vi "Configure Measurement Cursors.vi"(11 "State in":T1={"Graph Visible Items"={"Plot Legend"=FALSE, "Scale Legend"=FALSE, "Graph Palette"=FALSE, "Cursor Legend"=FALSE, "X Scrollbar"=FALSE}, "View Table"=FALSE, "Table Visible Items"={"Vertical Scrollbar"=FALSE, "Horizontal Scrollbar"=FALSE, "Row Headers"=FALSE, "Column Headers"=FALSE, "Vertical Lines"=FALSE, "Horizontal Lines"=FALSE}, "Header Font"={"Font Name"="", "Size"=0, "Bold"=FALSE, "Italic"=FALSE, "Underline"=FALSE, "Strikeout"=FALSE, "Color"=0}, "Cell Font"={"Font Name"="", "Size"=0, "Bold"=FALSE, "Italic"=FALSE, "Underline"=FALSE, "Strikeout"=FALSE, "Color"=0}, "Description and Tip..."={"Description"="", "Tip"=""}, "Moveable Splitter Position"=0, "Measurement Cursor Configuration"={"XY"={"enable XY"=FALSE, "Position (X)"=[], "Type"=enum."Absolute", "Y reference"=0.0, "color"=0}, "band"={"enable band"=FALSE, "B1"=0.0, "B2"=0.0, "Fixed bandwidth (B2-B1)"=0.0, "B1 color"=0, "B2 color"=0}, "harmonic"={"enable harmonics"=FALSE, "X reference (1X)"=0.0, "Maximum"=0, "Subset"=enum."All", "1X color"=0, "MX color"=0}, "sideband"={"enable sideband"=FALSE, "X center (C)"=0.0, "Sidebands"=0, "X spacing (s)"=0.0, "Center color"=0, "Sideband color"=0}}, "Cursors"={"List"=[], "Tags"=[]}, "X Increment"=0.0, "X Scale"={"Label Visible"=FALSE, "Label Text"="", "Mapping Mode"=0, "Format String"=""}, "Y Scale"={"Label Visible"=FALSE, "Label Text"="", "Mapping Mode"=0, "Format String"=""}, "Colors"={"background"=16777215, "major grid"=8355711, "minor grid"=12632256, "font"=0}, "desired spectrum view"={"scaling"={"linear/dB"=enum."no change", "dB reference"=0.0, "power/magnitude"=enum."no change", "view"=enum."no change"}, "spectral density"=enum."no change"}, "Plot Color Wheel"=[3381759, 32768, 982784, 4375295, 13827953, 13457919, 16757522, 4343295, 16728758, 12095254], "Plots"=[], "registered user events"=variant, "Lock 1X to Peak"=FALSE, "spectrum component"=32, "phase spectrum view"={"desired units"=0, "desired wrapping"=4}} caption="State" {"phase spectrum view"."desired wrapping" items=["No change", "Unwrap", "Wrap: -360 to 0", "Wrap: -270 to 90", "Wrap: -180 to 180", "Wrap: -90 to 270", "Wrap: 0 to 360", "Wrap: custom range"]; "phase spectrum view"."desired units" items=["No change", "Radians", "Degrees", "Cycles"]; "spectrum component" items=["Magnitude^2"=37, "Magnitude"=32, "Phase"=33, "Real"=34, "Imaginary"=35, "Coherence"=36, "Unknown"=99]; "Y Scale"."Mapping Mode" items=["Linear", "Logarithmic", "dB"]; "X Scale"."Mapping Mode" items=["Linear", "Logarithmic"]}) -> (1 "OK":bool, 3 "State out":T1={"Graph Visible Items"={"Plot Legend"=FALSE, "Scale Legend"=FALSE, "Graph Palette"=FALSE, "Cursor Legend"=FALSE, "X Scrollbar"=FALSE}, "View Table"=FALSE, "Table Visible Items"={"Vertical Scrollbar"=FALSE, "Horizontal Scrollbar"=FALSE, "Row Headers"=FALSE, "Column Headers"=FALSE, "Vertical Lines"=FALSE, "Horizontal Lines"=FALSE}, "Header Font"={"Font Name"="", "Size"=0, "Bold"=FALSE, "Italic"=FALSE, "Underline"=FALSE, "Strikeout"=FALSE, "Color"=0}, "Cell Font"={"Font Name"="", "Size"=0, "Bold"=FALSE, "Italic"=FALSE, "Underline"=FALSE, "Strikeout"=FALSE, "Color"=0}, "Description and Tip..."={"Description"="", "Tip"=""}, "Moveable Splitter Position"=0, "Measurement Cursor Configuration"={"XY"={"enable XY"=FALSE, "Position (X)"=[], "Type"=enum."Absolute", "Y reference"=0.0, "color"=0}, "band"={"enable band"=FALSE, "B1"=0.0, "B2"=0.0, "Fixed bandwidth (B2-B1)"=0.0, "B1 color"=0, "B2 color"=0}, "harmonic"={"enable harmonics"=FALSE, "X reference (1X)"=0.0, "Maximum"=0, "Subset"=enum."All", "1X color"=0, "MX color"=0}, "sideband"={"enable sideband"=FALSE, "X center (C)"=0.0, "Sidebands"=0, "X spacing (s)"=0.0, "Center color"=0, "Sideband color"=0}}, "Cursors"={"List"=[], "Tags"=[]}, "X Increment"=0.0, "X Scale"={"Label Visible"=FALSE, "Label Text"="", "Mapping Mode"=0, "Format String"=""}, "Y Scale"={"Label Visible"=FALSE, "Label Text"="", "Mapping Mode"=0, "Format String"=""}, "Colors"={"background"=16777215, "major grid"=8355711, "minor grid"=12632256, "font"=0}, "desired spectrum view"={"scaling"={"linear/dB"=enum."no change", "dB reference"=0.0, "power/magnitude"=enum."no change", "view"=enum."no change"}, "spectral density"=enum."no change"}, "Plot Color Wheel"=[3381759, 32768, 982784, 4375295, 13827953, 13457919, 16757522, 4343295, 16728758, 12095254], "Plots"=[], "registered user events"=variant, "Lock 1X to Peak"=FALSE, "spectrum component"=32, "phase spectrum view"={"desired units"=0, "desired wrapping"=4}} caption="State" {"phase spectrum view"."desired wrapping" items=["No change", "Unwrap", "Wrap: -360 to 0", "Wrap: -270 to 90", "Wrap: -180 to 180", "Wrap: -90 to 270", "Wrap: 0 to 360", "Wrap: custom range"]; "phase spectrum view"."desired units" items=["No change", "Radians", "Degrees", "Cycles"]; "spectrum component" items=["Magnitude^2"=37, "Magnitude"=32, "Phase"=33, "Real"=34, "Imaginary"=35, "Coherence"=36, "Unknown"=99]; "Y Scale"."Mapping Mode" items=["Linear", "Logarithmic", "dB"]; "X Scale"."Mapping Mode" items=["Linear", "Logarithmic"]})   [LabVIEW 2017, in "Spectrum with Cursors.xctl"]
doc: "Dialog for cursor configuration."
uses:
  <vilib>/addons/_XControls/Spectrum with Cursors/Spectrum with Cursors.xctl
  <vilib>/addons/_XControls/Spectrum with Cursors/Controls/State.ctl
  <vilib>/Utility/miscctls.llb/LVFontTypeDef.ctl
  <vilib>/addons/_XControls/Spectrum with Cursors/Controls/Measurement Cursor Configuration.ctl
  <vilib>/addons/_NISVFA/_Shared subVIs/Controls/NI Spectrum Component.ctl
panel:
  in  "XY color":u32(colorbox)
  in  "enable XY":bool
  in  "Type":enum16{"Absolute", "Relative"}(ring)
  in  "Position (i)":dbl[](array[numeric]) min=0.0 step=1.0
  in  "Y reference":dbl
  in  "B2 color":u32(colorbox)
  in  "B1 color":u32(colorbox)
  in  "Fixed bandwidth (B2-B1)":dbl=-1.0 caption="Fixed bandwidth"
  in  "enable band":bool
  in  "Stop (b2)":dbl=480.0
  in  "Start (b1)":dbl=20.0
  in  "1X color":u32(colorbox)
  in  "MX color":u32(colorbox)
  in  "enable harmonics":bool
  in  "Maximum (mX)":i32=10 min=2 max=99 step=1
  in  "X reference (1X)":dbl=60.0 min=0.001 step=1.0
  in  "Subset":enum16{"All", "Even", "Odd"}(ring)
  in  "Center color":u32(colorbox)
  in  "Sideband color":u32(colorbox)
  in  "Sidebands (sn)":i32=2 min=1 max=9 step=1
  in  "enable sideband":bool
  in  "X spacing (s)":dbl=60.0 min=0.0 step=1.0
  in  "X center (C)":dbl=8000.0 min=0.001 step=0.001
  in  "Cancel":bool
  in  "OK":bool
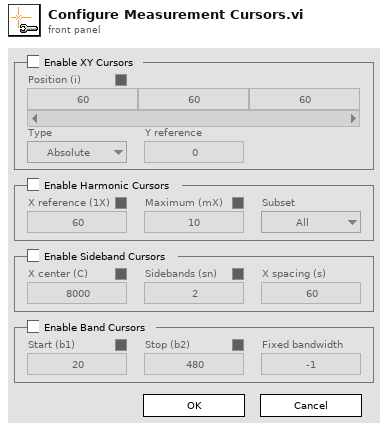
[diagram p1: front panel]
types:
  T1 = typedef "Spectrum with Cursors.xctl/State.ctl" = cluster{"Graph Visible Items":cluster{"Plot Legend":bool, "Scale Legend":bool, "Graph Palette":bool, "Cursor Legend":bool, "X Scrollbar":bool}, "View Table":bool, "Table Visible Items":cluster{"Vertical Scrollbar":bool, "Horizontal Scrollbar":bool, "Row Headers":bool, "Column Headers":bool, "Vertical Lines":bool, "Horizontal Lines":bool}, "Header Font":T2, "Cell Font":T2, "Description and Tip...":cluster{"Description":string, "Tip":string}, "Moveable Splitter Position":i32, "Measurement Cursor Configuration":T3, "Cursors":cluster{"List":cluster{"Name":string, "Color":u32, "Style":i32, "Point Style":u8, "Name Visible":bool, "Allow Drag":bool, "Cursor Mode":u32, "Plot":i32, "Index":i32, "Position":cluster{"X":dbl, "Y":dbl}, "X Scale":u32, "Y Scale":u32, "Watch Plots":i32[], "Watch All Plots":bool, "Plot Area":i32, "Label Offset":cluster{"X":dbl, "Y":dbl}}[], "Tags":variant[]}, "X Increment":dbl, "X Scale":cluster{"Label Visible":bool, "Label Text":string, "Mapping Mode":u8, "Format String":string}, "Y Scale":cluster{"Label Visible":bool, "Label Text":string, "Mapping Mode":u8, "Format String":string}, "Colors":cluster{"background":u32, "major grid":u32, "minor grid":u32, "font":u32}, "desired spectrum view":cluster{"scaling":cluster{"linear/dB":enum16{"no change", "linear", "dB"}, "dB reference":dbl, "power/magnitude":enum16{"no change", "power", "magnitude"}, "view":enum16{"no change", "rms", "peak", "peak-peak"}}, "spectral density":enum16{"no change", "spectrum", "spectral density"}}, "Plot Color Wheel":u32[], "Plots":cluster{"Name":string, "Line Color":u32, "Line Style":u8, "Line Width":u8, "Fill/Point Color":u32, "Point Style":u8, "Fill To":i16, "Interpolation":u8, "Anti-aliased":bool}[], "registered user events":variant, "Lock 1X to Peak":bool, "spectrum component":T4, "phase spectrum view":cluster{"desired units":u16, "desired wrapping":u16}}
  T2 = typedef "LVFontTypeDef.ctl" = cluster{"Font Name":string, "Size":u16, "Bold":bool, "Italic":bool, "Underline":bool, "Strikeout":bool, "Color":u32}
  T3 = typedef "Spectrum with Cursors.xctl/Measurement Cursor Configuration.ctl" = cluster{"XY":cluster{"enable XY":bool, "Position (X)":dbl[], "Type":enum16{"Absolute", "Relative"}, "Y reference":dbl, "color":u32}, "band":cluster{"enable band":bool, "B1":dbl, "B2":dbl, "Fixed bandwidth (B2-B1)":dbl, "B1 color":u32, "B2 color":u32}, "harmonic":cluster{"enable harmonics":bool, "X reference (1X)":dbl, "Maximum":i32, "Subset":enum16{"All", "Even", "Odd"}, "1X color":u32, "MX color":u32}, "sideband":cluster{"enable sideband":bool, "X center (C)":dbl, "Sidebands":i32, "X spacing (s)":dbl, "Center color":u32, "Sideband color":u32}}
  T4 = typedef "NI Spectrum Component.ctl" = u16
  T5 = cluster{"enable XY":bool, "Position (X)":dbl[], "Type":enum16{"Absolute", "Relative"}, "Y reference":dbl, "color":u32}
  T6 = cluster{"enable harmonics":bool, "X reference (1X)":dbl, "Maximum":i32, "Subset":enum16{"All", "Even", "Odd"}, "1X color":u32, "MX color":u32}
  T7 = cluster{"enable sideband":bool, "X center (C)":dbl, "Sidebands":i32, "X spacing (s)":dbl, "Center color":u32, "Sideband color":u32}
  T8 = cluster{"enable band":bool, "B1":dbl, "B2":dbl, "Fixed bandwidth (B2-B1)":dbl, "B1 color":u32, "B2 color":u32}
  T9 = enum8{"Enabled", "Disabled", "Disabled and Grayed Out"}
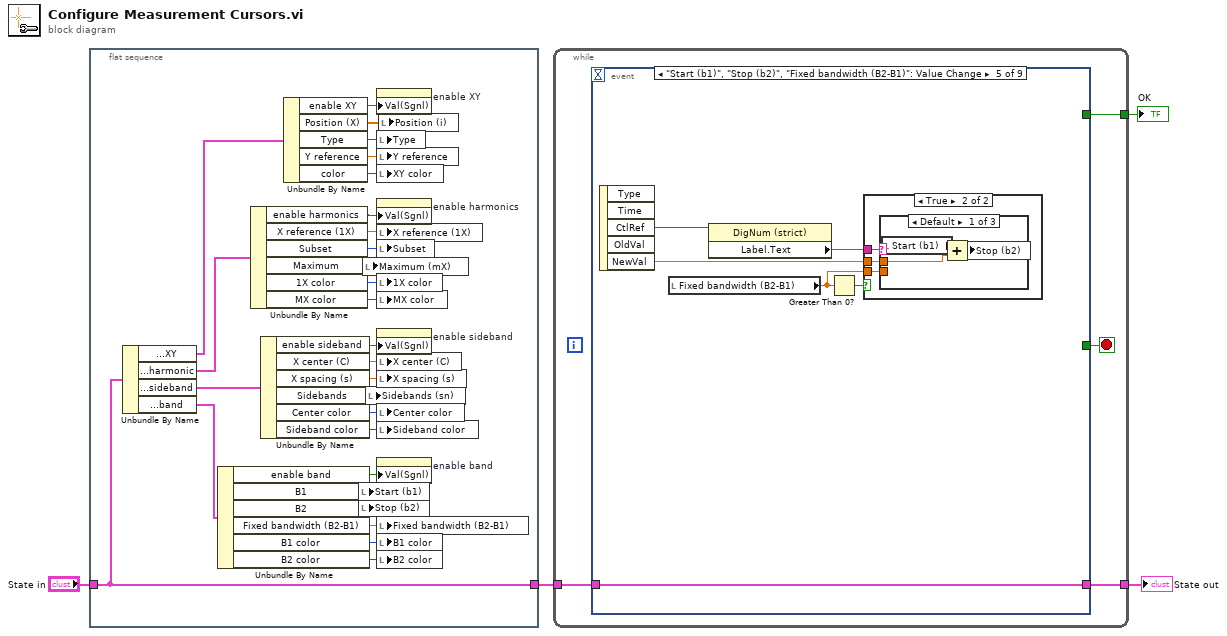
[diagram p0: block diagram]
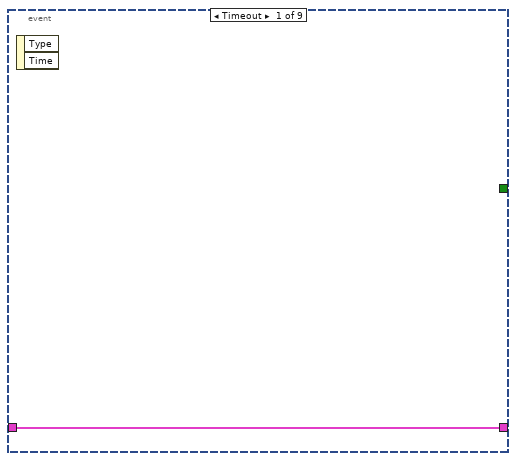
[diagram p2: hidden frame]
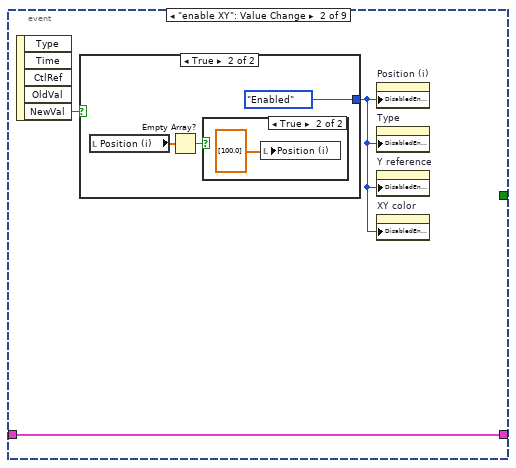
[diagram p3: hidden frame]
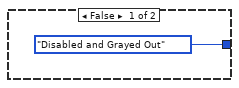
[diagram p4: hidden frame]
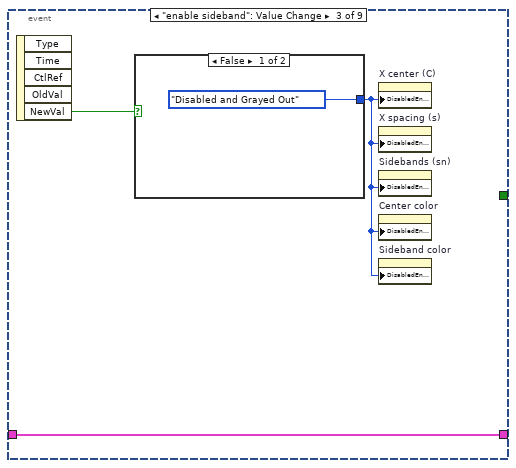
[diagram p6: hidden frame]
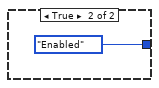
[diagram p7: hidden frame]
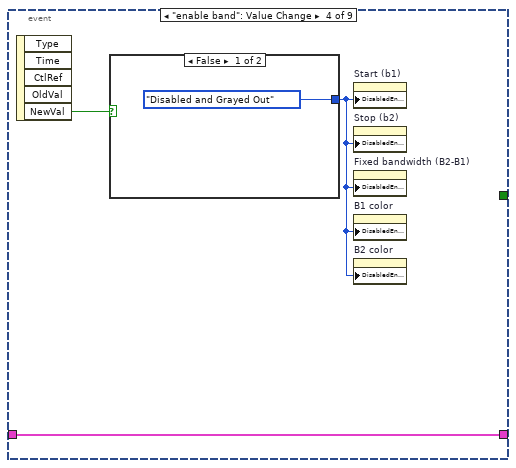
[diagram p8: hidden frame]
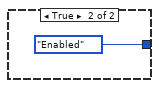
[diagram p9: hidden frame]
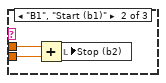
[diagram p11: hidden frame]
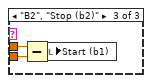
[diagram p12: hidden frame]
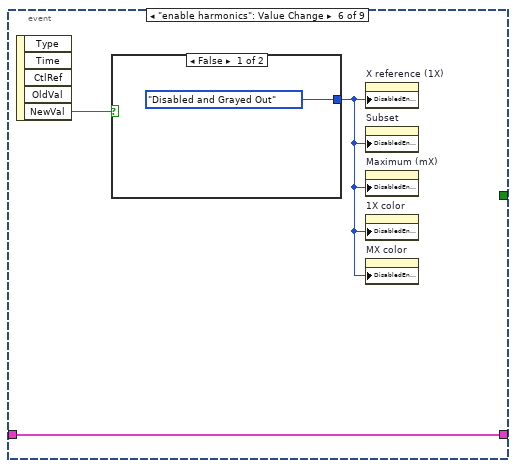
[diagram p13: hidden frame]
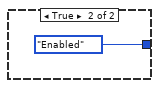
[diagram p14: hidden frame]
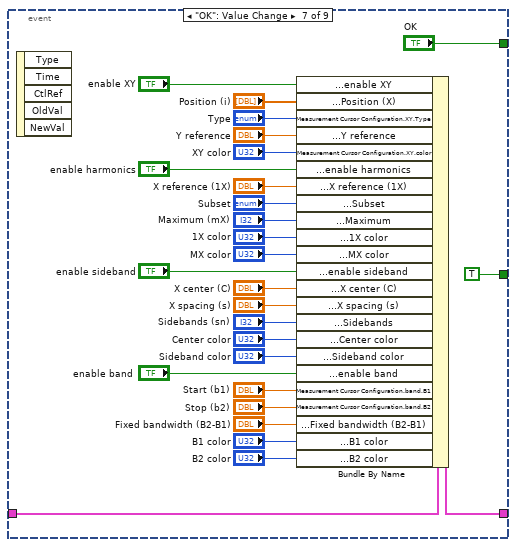
[diagram p15: hidden frame]
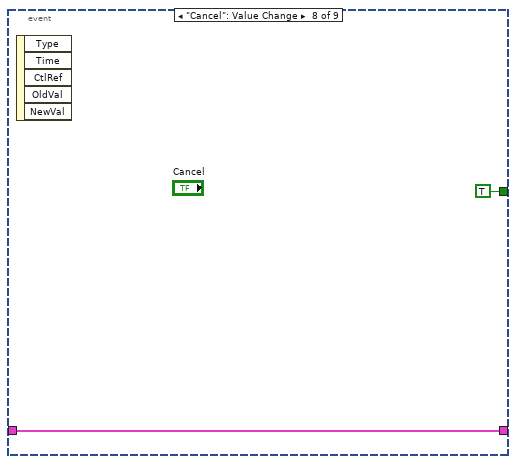
[diagram p16: hidden frame]
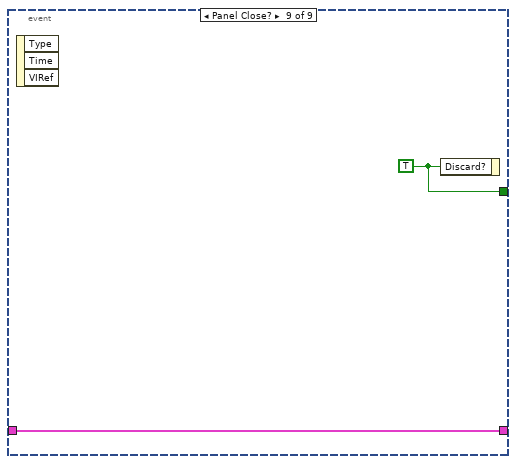
[diagram p17: hidden frame]
diagram:
  n1 = flat-sequence {
    tunnel: "State in" -> [w16]
    tunnel: [w16] -> w2
    frame #0 {
      n2 = Unbundle By Name(w16) -> ("Measurement Cursor Configuration.XY"=w32:T5, "Measurement Cursor Configuration.harmonic"=w28:T6, "Measurement Cursor Configuration.sideband"=w24:T7, "Measurement Cursor Configuration.band"=w20:T8)
      n3 = Unbundle By Name(w20) -> ("enable band"=w12:bool, "B1"=w19:dbl, "B2"=w18:dbl, "Fixed bandwidth (B2-B1)"=w17:dbl, "B1 color"=w6:u32, "B2 color"=w5:u32)
      n4 = Unbundle By Name(w28) -> ("enable harmonics"=w14:bool, "X reference (1X)"=w27:dbl, "Subset"=w26:enum16{"All", "Even", "Odd"}, "Maximum"=w25:i32, "1X color"=w10:u32, "MX color"=w9:u32)
      n5 = Unbundle By Name(w24) -> ("enable sideband"=w13:bool, "X center (C)"=w23:dbl, "X spacing (s)"=w22:dbl, "Sidebands"=w21:i32, "Center color"=w8:u32, "Sideband color"=w7:u32)
      n6 = Unbundle By Name(w32) -> ("enable XY"=w15:bool, "Position (X)"=w31:dbl[], "Type"=w30:enum16{"Absolute", "Relative"}, "Y reference"=w29:dbl, "color"=w11:u32)
      n7 = local write "Start (b1)"(w19) -> ()
      n8 = local write "Stop (b2)"(w18) -> ()
      n9 = local write "Maximum (mX)"(w25) -> ()
      n10 = local write "Sidebands (sn)"(w21) -> ()
      n11 = property on="enable XY" class="Bool (strict)"("Val(Sgnl)"=w15) -> ()  [unwired: 2 in, 2 out]
      n12 = local write "Type"(w30) -> ()
      n13 = local write "Y reference"(w29) -> ()
      n14 = local write "XY color"(w11) -> ()
      n15 = property on="enable harmonics" class="Bool (strict)"("Val(Sgnl)"=w14) -> ()  [unwired: 2 in, 2 out]
      n16 = local write "X reference (1X)"(w27) -> ()
      n17 = local write "Subset"(w26) -> ()
      n18 = local write "1X color"(w10) -> ()
      n19 = local write "MX color"(w9) -> ()
      n20 = property on="enable sideband" class="Bool (strict)"("Val(Sgnl)"=w13) -> ()  [unwired: 2 in, 2 out]
      n21 = local write "X center (C)"(w23) -> ()
      n22 = local write "X spacing (s)"(w22) -> ()
      n23 = local write "Center color"(w8) -> ()
      n24 = local write "Sideband color"(w7) -> ()
      n25 = property on="enable band" class="Bool (strict)"("Val(Sgnl)"=w12) -> ()  [unwired: 2 in, 2 out]
      n26 = local write "Fixed bandwidth (B2-B1)"(w17) -> ()
      n27 = local write "B1 color"(w6) -> ()
      n28 = local write "B2 color"(w5) -> ()
      n29 = local write "Position (i)"(w31) -> ()
    }
  }
  n30 = while {
    tunnel: w2 -> [w34]
    tunnel: [w35] -> w4
    tunnel: [w33] -> w1
    stop <- w36 stop-if-true
    n31 = event shown="[4] \"Start (b1)\", \"Stop (b2)\", \"Fixed bandwidth (B2-B1)\": Value Change" {
      selector: _ -> [_ _ _ _ _ _ _ _ _]
      dyn-events: _ -> [_ _ _ _ _ _ _ _ _]
      timeout: _ -> [_ _ _ _ _ _ _ _ _]
      tunnel: [_ _ _ _ _ _ TRUE TRUE w108] -> w36
      tunnel: [w37 w39 w47 w52 w61 w75 w90 w106 w109] -> w35
      tunnel: w34 -> [w37 w39 w47 w52 w61 w75 w91 w106 w109]
      tunnel: [_ _ _ _ _ _ "OK" _ _] -> w33
      event Timeout {
        n32 = event-data() -> ()  [unwired: 1 in, 2 out]
      }
      event "enable XY": Value Change {
        n33 = event-data() -> ("NewVal"=w40:bool)  [unwired: 1 in, 4 out]
        n34 = case shown="True" w40 {
          tunnel: [T9."Disabled and Grayed Out" ("Disabled") T9."Enabled" ("Disabled")] -> w38
          frame False {
          }
          frame True {
            n35 = local read "Position (i)"() -> (w43:dbl[])
            n36 = Empty Array?(array=w43) -> (empty?=w42:bool)
            n37 = case shown="True" w42 {
              frame False {
              }
              frame True {
                n38 = local write "Position (i)"(dbl[] [100.0] ("Position (i)")) -> ()
              }
            }
          }
        }
        n39 = property on="Position (i)" class="Arr (strict)"("DisabledEnum"=w38) -> ()  [unwired: 2 in, 2 out]
        n40 = property on="Type" class="Enum (strict)"("DisabledEnum"=w38) -> ()  [unwired: 2 in, 2 out]
        n41 = property on="Y reference" class="DigNum (strict)"("DisabledEnum"=w38) -> ()  [unwired: 2 in, 2 out]
        n42 = property on="XY color" class="ColBox"("DisabledEnum"=w38) -> ()  [unwired: 2 in, 2 out]
      }
      event "enable sideband": Value Change {
        n43 = event-data() -> ("NewVal"=w48:bool)  [unwired: 1 in, 4 out]
        n44 = case shown="False" w48 {
          tunnel: [T9."Disabled and Grayed Out" ("Disabled") T9."Enabled" ("Disabled")] -> w46
          frame False {
          }
          frame True {
          }
        }
        n45 = property on="X center (C)" class="DigNum (strict)"("DisabledEnum"=w46) -> ()  [unwired: 2 in, 2 out]
        n46 = property on="X spacing (s)" class="DigNum (strict)"("DisabledEnum"=w46) -> ()  [unwired: 2 in, 2 out]
        n47 = property on="Sidebands (sn)" class="DigNum (strict)"("DisabledEnum"=w46) -> ()  [unwired: 2 in, 2 out]
        n48 = property on="Center color" class="ColBox"("DisabledEnum"=w46) -> ()  [unwired: 2 in, 2 out]
        n49 = property on="Sideband color" class="ColBox"("DisabledEnum"=w46) -> ()  [unwired: 2 in, 2 out]
      }
      event "enable band": Value Change {
        n50 = event-data() -> ("NewVal"=w53:bool)  [unwired: 1 in, 4 out]
        n51 = case shown="False" w53 {
          tunnel: [T9."Disabled and Grayed Out" ("Disabled") T9."Enabled" ("Disabled")] -> w51
          frame False {
          }
          frame True {
          }
        }
        n52 = property on="Start (b1)" class="DigNum (strict)"("DisabledEnum"=w51) -> ()  [unwired: 2 in, 2 out]
        n53 = property on="Stop (b2)" class="DigNum (strict)"("DisabledEnum"=w51) -> ()  [unwired: 2 in, 2 out]
        n54 = property on="Fixed bandwidth (B2-B1)" class="DigNum (strict)"("DisabledEnum"=w51) -> ()  [unwired: 2 in, 2 out]
        n55 = property on="B1 color" class="ColBox"("DisabledEnum"=w51) -> ()  [unwired: 2 in, 2 out]
        n56 = property on="B2 color" class="ColBox"("DisabledEnum"=w51) -> ()  [unwired: 2 in, 2 out]
      }
      event "Start (b1)", "Stop (b2)", "Fixed bandwidth (B2-B1)": Value Change {
        n57 = event-data() -> ("CtlRef"=w60:refnum<vi>, "NewVal"=w58:dbl)  [unwired: 1 in, 3 out]
        n58 = local read "Fixed bandwidth (B2-B1)"() -> (w56:dbl)
        n59 = property class="DigNum (strict)"(reference=w60) -> ("Label.Text"=w59:string)  [unwired: 1 in, 2 out]
        n60 = Greater Than 0?(x=w56) -> (x > 0?=w57:bool)
        n61 = case shown="True" w57 {
          tunnel: w59 -> [_ w64]
          tunnel: w58 -> [_ w63]
          tunnel: w56 -> [_ w62]
          frame False {
          }
          frame True {
            n62 = case shown="Default" w64 {
              tunnel: w63 -> [w67 w70 w73]
              tunnel: w62 -> [_ w69 w72]
              frame Default {
                n63 = local read "Start (b1)"() -> (w66:dbl)
                n64 = Add(x=w66, y=w67) -> (x+y=w65:dbl)
                n65 = local write "Stop (b2)"(w65) -> ()
              }
              frame "B1", "Start (b1)" {
                n66 = Add(x=w70, y=w69) -> (x+y=w68:dbl)
                n67 = local write "Stop (b2)"(w68) -> ()
              }
              frame "B2", "Stop (b2)" {
                n68 = Subtract(x=w73, y=w72) -> (x-y=w71:dbl)
                n69 = local write "Start (b1)"(w71) -> ()
              }
            }
          }
        }
      }
      event "enable harmonics": Value Change {
        n70 = event-data() -> ("NewVal"=w76:bool)  [unwired: 1 in, 4 out]
        n71 = case shown="False" w76 {
          tunnel: [T9."Disabled and Grayed Out" ("Disabled") T9."Enabled" ("Disabled")] -> w74
          frame False {
          }
          frame True {
          }
        }
        n72 = property on="X reference (1X)" class="DigNum (strict)"("DisabledEnum"=w74) -> ()  [unwired: 2 in, 2 out]
        n73 = property on="Subset" class="Enum (strict)"("DisabledEnum"=w74) -> ()  [unwired: 2 in, 2 out]
        n74 = property on="Maximum (mX)" class="DigNum (strict)"("DisabledEnum"=w74) -> ()  [unwired: 2 in, 2 out]
        n75 = property on="1X color" class="ColBox"("DisabledEnum"=w74) -> ()  [unwired: 2 in, 2 out]
        n76 = property on="MX color" class="ColBox"("DisabledEnum"=w74) -> ()  [unwired: 2 in, 2 out]
      }
      event "OK": Value Change {
        n77 = event-data() -> ()  [unwired: 1 in, 5 out]
        n78 = Bundle By Name(cluster=w91, "Measurement Cursor Configuration.XY.enable XY"="enable XY", "Measurement Cursor Configuration.XY.Position (X)"="Position (i)", "Measurement Cursor Configuration.XY.Type"="Type", "Measurement Cursor Configuration.XY.Y reference"="Y reference", "Measurement Cursor Configuration.XY.color"="XY color", "Measurement Cursor Configuration.harmonic.enable harmonics"="enable harmonics", "Measurement Cursor Configuration.harmonic.X reference (1X)"="X reference (1X)", "Measurement Cursor Configuration.harmonic.Subset"="Subset", "Measurement Cursor Configuration.harmonic.Maximum"="Maximum (mX)", "Measurement Cursor Configuration.harmonic.1X color"="1X color", "Measurement Cursor Configuration.harmonic.MX color"="MX color", "Measurement Cursor Configuration.sideband.enable sideband"="enable sideband", "Measurement Cursor Configuration.sideband.X center (C)"="X center (C)", "Measurement Cursor Configuration.sideband.X spacing (s)"="X spacing (s)", "Measurement Cursor Configuration.sideband.Sidebands"="Sidebands (sn)", "Measurement Cursor Configuration.sideband.Center color"="Center color", "Measurement Cursor Configuration.sideband.Sideband color"="Sideband color", "Measurement Cursor Configuration.band.enable band"="enable band", "Measurement Cursor Configuration.band.B1"="Start (b1)", "Measurement Cursor Configuration.band.B2"="Stop (b2)", "Measurement Cursor Configuration.band.Fixed bandwidth (B2-B1)"="Fixed bandwidth (B2-B1)", "Measurement Cursor Configuration.band.B1 color"="B1 color", "Measurement Cursor Configuration.band.B2 color"="B2 color") -> (w90:T1)
      }
      event "Cancel": Value Change {
        n79 = event-data() -> ()  [unwired: 1 in, 5 out]
      }
      event Panel Close? {
        w108 = TRUE
        n80 = event-data() -> ()  [unwired: 1 in, 3 out]
        n81 = event-data("Discard?"=w108) -> ()  [unwired: 1 in, 1 out]
      }
    }
  }
  "State out" <- w4
  "OK" <- w1
